vi "EditorThumbnail resizePanel.vi"(8 "error in (no error)":errorcluster, 11 "EditorThumbnail in":refnum<class "EditorThumbnail.lvclass">) -> (0 "error out":errorcluster, 3 "EditorThumbnail out":refnum<class "EditorThumbnail.lvclass">)   [LabVIEW 2018, in "EditorThumbnail.lvclass"]
uses:
  EditorThumbnail.lvclass
  EditorThumbnail.lvclass/EditorThumbnail.ctl
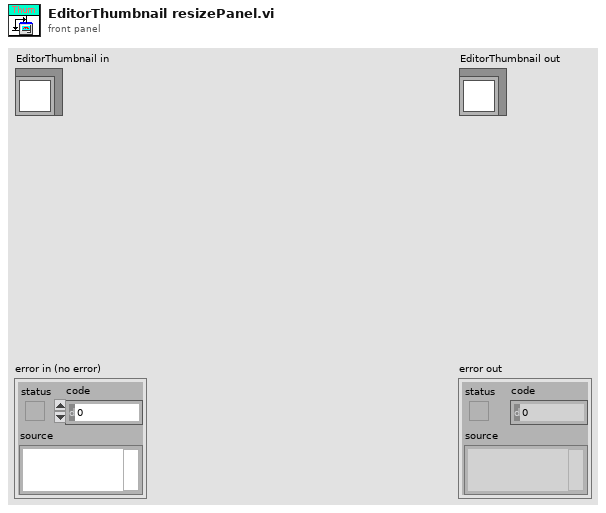
[diagram p1: front panel]
types:
  T1 = cluster{"index":u32, "data":cluster{"xdata":dbl[], "ydata":sgl[]}[], "peak":dbl[], "picture":picture}[]
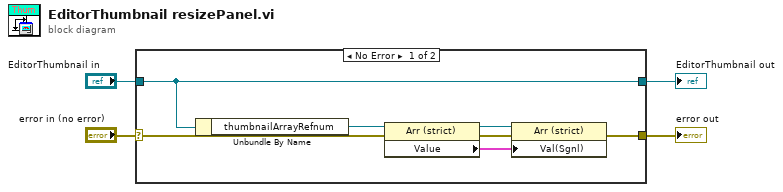
[diagram p0: block diagram]
diagram:
  n1 = case shown="No Error" "error in (no error)" {
    selector: "error in (no error)" -> [w6 w13]
    tunnel: [w5 w13] -> w3
    tunnel: [w11 w12] -> w1
    tunnel: "EditorThumbnail in" -> [w11 w12]
    frame No Error {
      n2 = Unbundle By Name(w11) -> ("thumbnailArrayRefnum"=w10:refnum<vi>)
      n3 = property class="Arr (strict)"(reference=w10, error in=w6) -> (reference out=w9:refnum<vi>, error out=w8:errorcluster, "Value"=w7:T1)
      n4 = property class="Arr (strict)"(reference=w9, error in=w8, "Val(Sgnl)"=w7) -> (error out=w5:errorcluster)  [unwired: 1 out]
    }
    frame Error {
    }
  }
  "error out" <- w3
  "EditorThumbnail out" <- w1
